vi "FM Ch Read Frm.vi"(6 "pReturned":u32, 8 "pBuffer":u8[](array[numeric]), 9 "BufSize":u32, 10 "Channel":u8, 11 "devId":i32) -> (0 "pBuffer out":u8[](array[numeric]), 2 "devId out":i32, 3 "function return":i32, 4 "pReturned out":u32)   [LabVIEW 2013, in "CHR34XXX.lvlib"]
doc: "DLL BOOL __stdcall CHR34XXX_FM_Ch_RxMode(IN int devId,IN BYTE Channel,IN BYTE RxMode); DLL BOOL __stdcall CHR34XXX_FM_Ch_RxFrmCount(IN int devId,IN BYTE Channel,OUT DWORD *FrmCnt); DLL BOOL __stdcall CHR34XXX_FM_Ch_ReadFrm(IN int devId,IN BYTE Channel,IN DWORD BufSize,OUT BYTE *pBuffer,OUT DWORD *pReturned);"
uses:
  CHR34XXX.lvlib
  CHR34XXX.dll
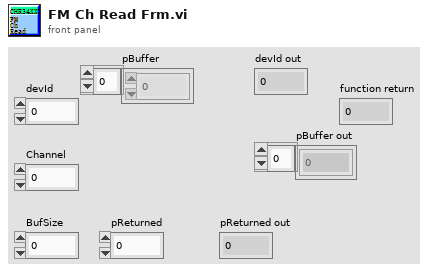
[diagram p1: front panel]
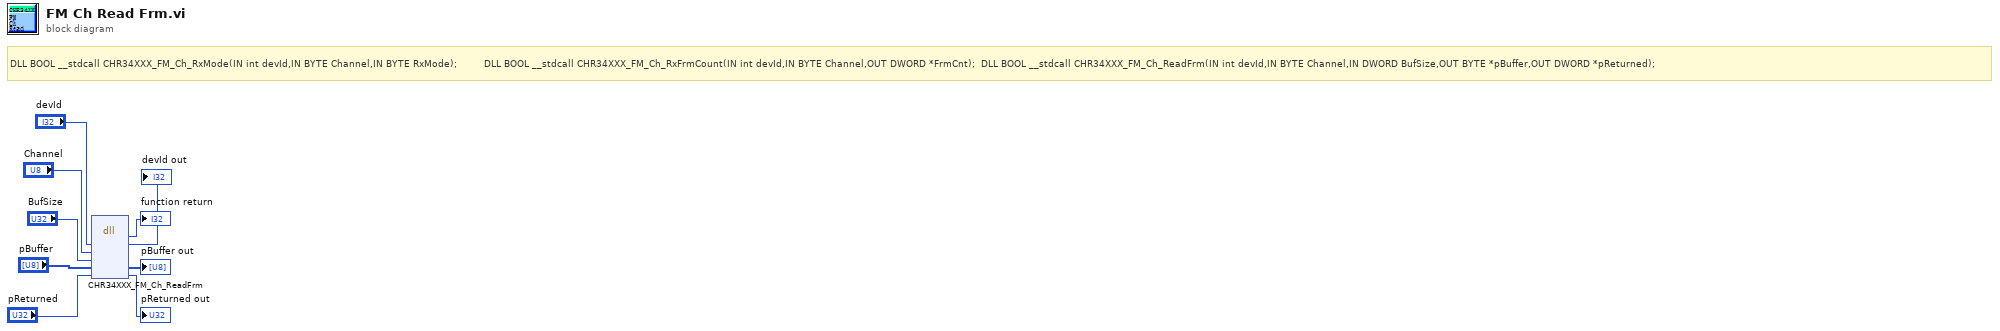
[diagram p0: block diagram]
diagram:
  # "DLL BOOL __stdcall CHR34XXX_FM_Ch_RxMode(IN int devId,IN BYTE Channel,IN BYTE RxMode);         DLL BOOL __stdcall CHR34XXX_FM_Ch_RxFrmCount(IN int devId,IN BYTE Channel,OUT DWORD *FrmCnt);  DLL BOOL __stdcall CHR34XXX_FM_Ch_ReadFrm(IN int devId,IN BYTE Channel,IN DWORD BufSize,OUT BYTE *pBuffer,OUT DWORD *pReturned);"
  n1 = dll-call lib="C:/Users/Administrator/Desktop/CHR34XXX_lv/lv_lib/CHR34XXX.*" fn="CHR34XXX_FM_Ch_ReadFrm"("devId"="devId", "Channel"="Channel", "BufSize"="BufSize", "pBuffer"="pBuffer", "pReturned"="pReturned") -> ("返回类型"=→"function return":i32, "devId"=→"devId out":i32, "pBuffer"=→"pBuffer out":u8[], "pReturned"=→"pReturned out":u32)  [unwired: 5 in, 2 out]
